vi "1_Boolean_Adder(Training).vi"() -> ()   [LabVIEW 2020]
uses:
  <vilib>/Ngene/DeepLTK/Toolkit/NN_Train/Controls/NN_Train_Params.ctl
  <vilib>/Ngene/DeepLTK/Toolkit/NN_Train/Controls/NN_Train_Optimizer.ctl
  <vilib>/Ngene/DeepLTK/Toolkit/NN_Train/Controls/NN_Train_Data_Sampling.ctl
  <vilib>/Ngene/DeepLTK/Toolkit/NN_Train/Controls/NN_LR_Policy_Cfg.ctl
  <vilib>/Ngene/DeepLTK/Toolkit/NN_Train/Controls/NN_LR_Policy_Type.ctl
  <vilib>/Ngene/DeepLTK/Toolkit/NN_Train/Controls/NN_Train_Session_Data.ctl
  <vilib>/Ngene/DeepLTK/Toolkit/NN_Data/API/DataSet_Types/NN_DataSet(In1D_Out1D).ctl
  <vilib>/Ngene/DeepLTK/Toolkit/NN_Data/API/DataRef_Types/NN_Data_ref(2D_SGL).ctl
  <vilib>/Ngene/DeepLTK/Toolkit/NN_Data/API/DataRef_Types/NN_Data_ref(1D_I32).ctl
  <vilib>/Ngene/DeepLTK/Toolkit/NN_Network/Controls/NN_Device.ctl
  <vilib>/Ngene/DeepLTK/Toolkit/NN_Layers/Layers/FC/Controls/NN_Layer_Config(FC).ctl
  <vilib>/Ngene/DeepLTK/Toolkit/NN_Activations/Controls/NN_Activation_Type.ctl
  <vilib>/Ngene/DeepLTK/Toolkit/NN_Layers/Controls/NN_Layer_Init_Params.ctl
  <vilib>/Ngene/DeepLTK/Toolkit/NN_Layers/Controls/NN_Layer_Weight_Init_Type.ctl
  <vilib>/Ngene/DeepLTK/Toolkit/NN_Network/Controls/NN_Save_Before_Destroy_Options.ctl
  <vilib>/Ngene/DeepLTK/Toolkit/NN_Layers/Layers/Input/Controls/NN_Layer_Config(Input1D).ctl
  <vilib>/Ngene/DeepLTK/Toolkit/NN_Layers/Layers/Input/NN_Layer_Create(Input1D).vi
  <vilib>/Ngene/DeepLTK/Toolkit/NN_Layers/Layers/FC/NN_Layer_Create(FC).vi
  <vilib>/Ngene/DeepLTK/Toolkit/NN_Train/Loss_Functions/NN_Set_Loss(MSE).vi
  <vilib>/Ngene/DeepLTK/Toolkit/NN_Network/subVIs/NN_Predict/NN_Predict(In1D_Out1D).vi
  <vilib>/Ngene/DeepLTK/Toolkit/Deep_Learning_Toolkit_by_Ngene.lvlib
  <vilib>/ptbypt/NI_PtbyPt.lvlib
panel:
  out "Loss Chart":cluster{"mean":dbl, "Error Rate":dbl}(graph)={"mean"=0.0016345112270209938, "Error Rate"=0.0}
  in  "stop":bool
  out "Loop Time":dbl=0.31297880000056466 format="%#_4p"
  out "Error Rate":dbl format="%#_6p"
  out "Loss":sgl=0.0016345113 format="%#_6p"
  in  "?":bool=TRUE
  out "Session Data":T1={"Epochs"=6.9160156, "Tot_Iter"=7082, "LR"=0.05, "LR_iter"=7083}
  in  "LR_Decay_Params":T2={"Policy_Type"=enum."Step", "LR0"=0.09999999999999999, "k"=5.0, "WarmUp_Policy"=enum."Ramp", "WarmUp_Iter"=1000, "WarmUp_Ratio"=1000.0} {"WarmUp_Ratio" min=1; "WarmUp_Iter" min=1; "LR0" format="%.7f"}
  in  "NN_Train_Params":T4={"Optimizer"=enum."SGD", "Beta_1"=0.9, "Beta_2"=0.0, "Weight Decay(L1)"=1e-08, "Weight Decay(L2)"=1e-08, "Data_Sampling"=enum."Random"}
  # "Overview: Demonstrates the usage of Deep Learning Toolkit for solving Boolean Adder problem.\nRequirements: DeepLTK - Deep Learning Toolkit for LabVIEW (https://www.ngene.co/deep-learning-toolkit-for-labview)\nInstructions:\n1. Run the VI.\n2. Observe how the training loss is decreasing.\n3. Observe the training speed.\n4. Press the Stop Train button when the curve stops decreasing.\nMore Examples:  https://github.com/ngenehub/deepltk_examples"
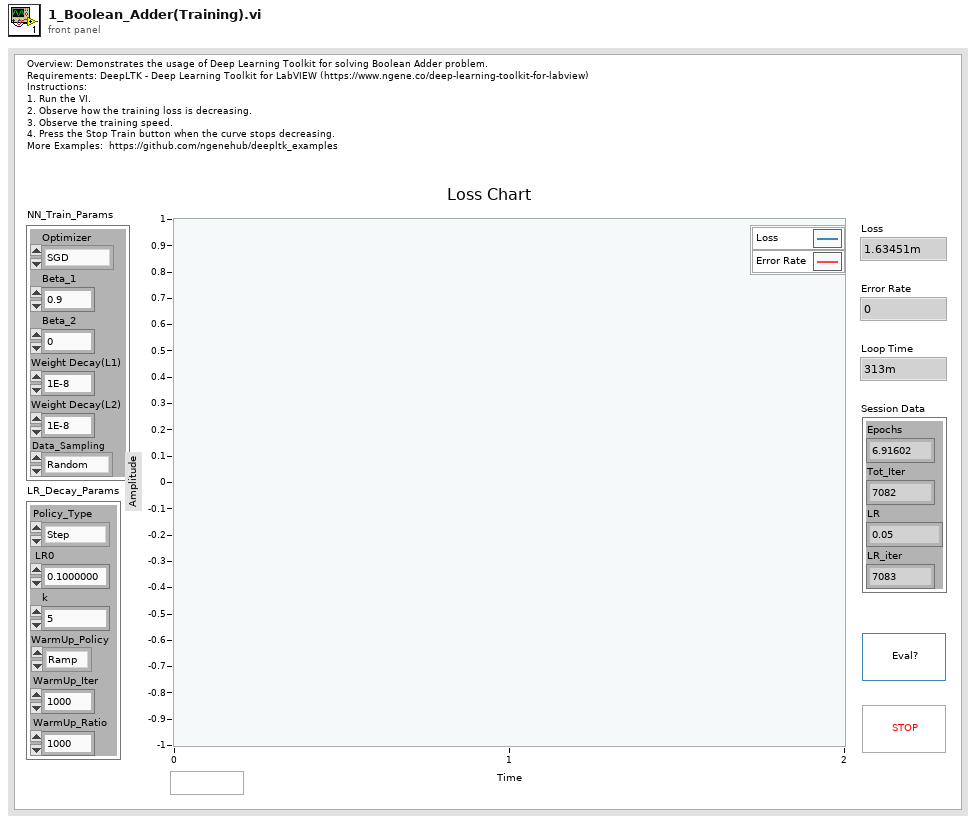
[diagram p1: front panel]
types:
  T1 = typedef "Deep_Learning_Toolkit_by_Ngene.lvlib/NN_Train_Session_Data.ctl" = cluster{"Epochs":sgl, "Tot_Iter":i32, "LR":sgl, "LR_iter":i32}
  T2 = typedef "Deep_Learning_Toolkit_by_Ngene.lvlib/NN_LR_Policy_Cfg.ctl" = cluster{"Policy_Type":T3, "LR0":dbl, "k":sgl, "WarmUp_Policy":enum16{"Step", "Ramp"}, "WarmUp_Iter":i32, "WarmUp_Ratio":sgl}
  T3 = typedef "Deep_Learning_Toolkit_by_Ngene.lvlib/NN_LR_Policy_Type.ctl" = enum16{"Manual", "Step", "Exp", "1/t"}
  T4 = typedef "Deep_Learning_Toolkit_by_Ngene.lvlib/NN_Train_Params.ctl" = cluster{"Optimizer":T5, "Beta_1":sgl, "Beta_2":sgl, "Weight Decay(L1)":sgl, "Weight Decay(L2)":sgl, "Data_Sampling":T6}
  T5 = typedef "Deep_Learning_Toolkit_by_Ngene.lvlib/NN_Train_Optimizer.ctl" = enum16{"SGD", "Adam", "Adagrad", "Adadelta", "RMSProp", "Nesterov"}
  T6 = typedef "Deep_Learning_Toolkit_by_Ngene.lvlib/NN_Train_Data_Sampling.ctl" = enum16{"Random", "Sequential"}
  T7 = typedef "Deep_Learning_Toolkit_by_Ngene.lvlib/NN_DataSet(In1D_Out1D).ctl" = cluster{"Inputs Ref.":T8, "Outputs Ref.":T8, "Dims_In":i32, "Dataset_Size":i32, "Outputs_idx Ref.":T9, "Dims_Out":i32, "Labels":string[], "File Paths":path[]}
  T8 = typedef "Deep_Learning_Toolkit_by_Ngene.lvlib/NN_Data_ref(2D_SGL).ctl" = refnum<data-value>
  T9 = typedef "Deep_Learning_Toolkit_by_Ngene.lvlib/NN_Data_ref(1D_I32).ctl" = refnum<data-value>
  T10 = typedef "Deep_Learning_Toolkit_by_Ngene.lvlib/NN_Layer_Config(FC).ctl" = cluster{"Name":string, "Size":i32, "BN":bool, "Activation":T11, "Init_Params":T12, "Custom_Params":string}
  T11 = typedef "Deep_Learning_Toolkit_by_Ngene.lvlib/NN_Activation_Type.ctl" = enum16{"Sigmoid", "ReLU", "LReLU", "ReLU6", "tanh", "Swish", "Mish", "None"}
  T12 = typedef "Deep_Learning_Toolkit_by_Ngene.lvlib/NN_Layer_Init_Params.ctl" = cluster{"Init_Type":T13, "Value":sgl}
  T13 = typedef "Deep_Learning_Toolkit_by_Ngene.lvlib/NN_Layer_Weight_Init_Type.ctl" = enum16{"Const", "Uniform", "Gaussian", "Xavier"}
  T14 = typedef "Deep_Learning_Toolkit_by_Ngene.lvlib/NN_Device.ctl" = enum16{"CPU", "GPU"}
  T15 = typedef "Deep_Learning_Toolkit_by_Ngene.lvlib/NN_Save_Before_Destroy_Options.ctl" = cluster{"CFG?":bool, "Weights?":bool, "Render?":bool}
  T16 = typedef "Deep_Learning_Toolkit_by_Ngene.lvlib/NN_Layer_Config(Input1D).ctl" = cluster{"Name":string, "Size":i32}
  T17 = typedef "Deep_Learning_Toolkit_by_Ngene.lvlib/NN.ctl" = cluster{"Name":string, "No of Layers":i32, "mBatch":i32, "Layers":T18[], "Dimty":T19, "Dims_In":T20, "Dims_Out":T20, "Working_Dir":path, "Train?":bool, "Train_Params":T4, "LR_Update_Policy":T2, "Session Data":T1, "Ground_truth":T21, "NNg_hdls":T22, "NN_Device":T14, "GPU Id":i32, "Labels":string[], "Receptive Field":T23[], "Loss_Type":T24, "Loss_Cfg_Prms":variant}
  T18 = typedef "Deep_Learning_Toolkit_by_Ngene.lvlib/NN_Layer_ref.ctl" = refnum<data-value>
  T19 = typedef "Deep_Learning_Toolkit_by_Ngene.lvlib/NN_In_Out_Dim-ty.ctl" = enum8{"In1D_Out1D", "In3D_Out1D", "In3D_Out3D", "In3D_OutBBox"}
  T20 = typedef "Deep_Learning_Toolkit_by_Ngene.lvlib/NN_Dims(C,H,W).ctl" = cluster{"C":i32, "H":i32, "W":i32}
  T21 = typedef "Deep_Learning_Toolkit_by_Ngene.lvlib/NN_Ground_truth.ctl" = cluster{"Y":variant, "Y_idx":T9}
  T22 = typedef "Deep_Learning_Toolkit_by_Ngene.lvlib/nng_cuda_handles.ctl" = cluster{"cudnn":u64, "cublas":u64, "stream":u64, "curand":u64}
  T23 = typedef "Deep_Learning_Toolkit_by_Ngene.lvlib/NN_Dims(V,H).ctl" = cluster{"V":i32, "H":i32}
  T24 = typedef "Deep_Learning_Toolkit_by_Ngene.lvlib/NN_Loss_Type.ctl" = enum16{"None", "MSE", "CrossEntropy", "YOLO_v2"}
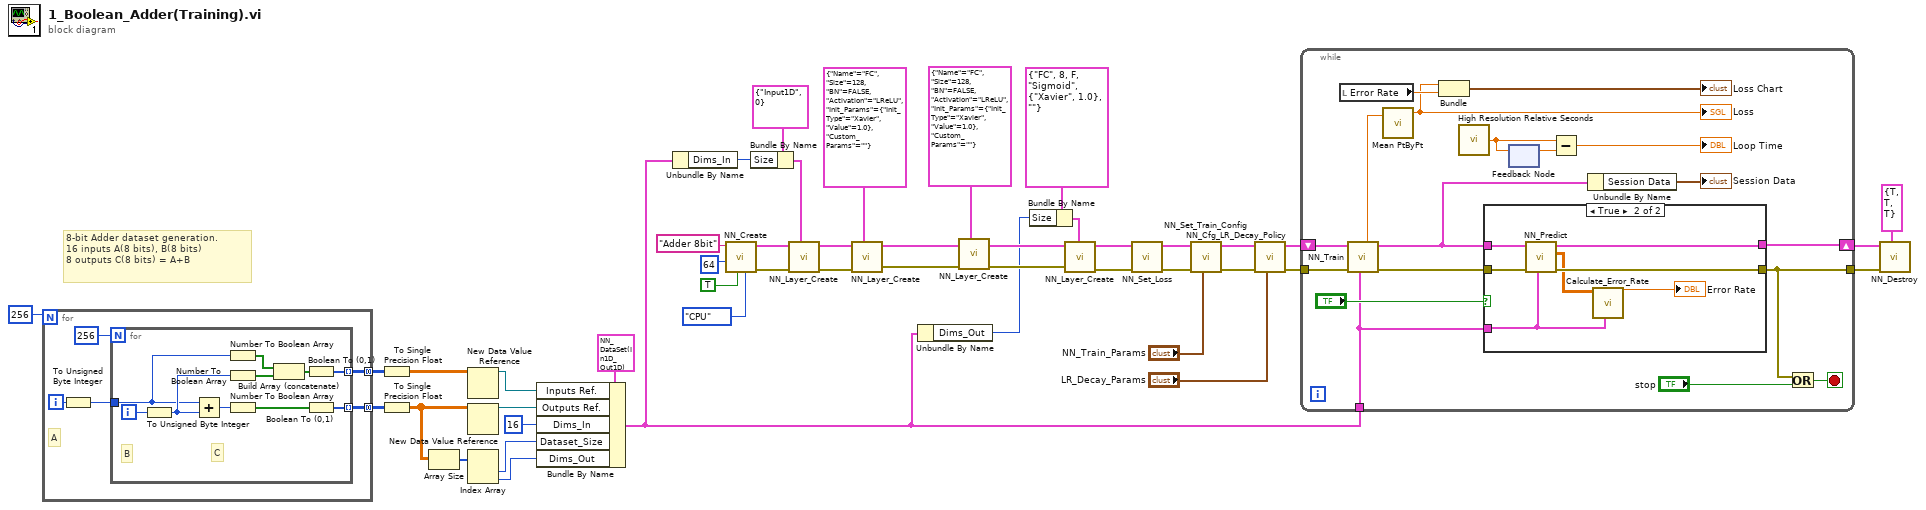
[diagram p0: block diagram]
diagram:
  # "8-bit Adder dataset generation.\n16 inputs A(8 bits), B(8 bits)\n8 outputs C(8 bits) = A+B"
  n1 = for {
    N: 256 -> [_]
    tunnel: [w50] -> w14 mode=concatenating
    tunnel: [w49] -> w13 mode=concatenating
    i -> [w48]
    # "A"
    n2 = To Unsigned Byte Integer(number=w48) -> (unsigned 8bit integer=w47:u8)
    n3 = for {
      N: 256 -> [_]
      tunnel: [w60] -> w49 mode=indexing
      tunnel: [w57] -> w50 mode=indexing
      tunnel: w47 -> [w54]
      i -> [w56]
      # "C"
      # "B"
      n4 = To Unsigned Byte Integer(number=w56) -> (unsigned 8bit integer=w55:u8)
      n5 = Add(x=w54, y=w55) -> (x+y=w58:u8)
      n6 = Number To Boolean Array(number=w54) -> (Boolean array=w52:bool[])
      n7 = Number To Boolean Array(number=w55) -> (Boolean array=w61:bool[])
      n8 = Number To Boolean Array(number=w58) -> (Boolean array=w59:bool[])
      n9 = Build Array (concatenate)(w52, w61) -> (w53:bool[])
      n10 = Boolean To (0,1)(Boolean=w53) -> (0, 1=w60:i16[])
      n11 = Boolean To (0,1)(Boolean=w59) -> (0, 1=w57:i16[])
    }
  }
  n12 = To Single Precision Float(number=w13) -> (single precision float=w7:sgl[][])
  n13 = To Single Precision Float(number=w14) -> (single precision float=w11:sgl[][])
  n14 = Array Size(array=w11) -> (size(s)=w10:i32[])
  n15 = New Data Value Reference(data value=w7) -> (data value reference=w16:refnum<data-value>)  [unwired: 1 in, 1 out]
  n16 = New Data Value Reference(data value=w11) -> (data value reference=w15:refnum<data-value>)  [unwired: 1 in, 1 out]
  n17 = Index Array(array=w10) -> (element #1=w9:i32, element #2=w8:i32)  [unwired: 2 in]
  n18 = Bundle By Name(cluster=T7 {"Inputs Ref."=refnum, "Outputs Ref."=refnum, "Dims_In"=0, "Dataset_Size"=0, "Outputs_idx Ref."=refnum, "Dims_Out"=0, "Labels"=[], "File Paths"=[]} ("Dataset(In1D_Out1D)"), "Inputs Ref."=w16, "Outputs Ref."=w15, "Dims_In"=16, "Dataset_Size"=w9, "Dims_Out"=w8) -> (w1:T7)
  n19 = Unbundle By Name(w1) -> ("Dims_In"=w2:i32)
  n20 = call <vilib>:"NN_Create.vi"("NN_Device"=NN_Device."CPU", "Train? (false)"=TRUE, "mBatch (1)"=64, "Name"="Adder 8bit") -> ("error out"=w43:errorcluster, "NN out"=w44:T17)  [unwired: 6 in]
  n21 = Bundle By Name(cluster=T16 {"Name"="Input1D", "Size"=0} ("Input1D_Cfg"), "Size"=w2) -> (w38:T16)
  n22 = call-poly <vilib>:"NN_Layer_Create.vi"("Input1D_Cfg"=w38, "error in (no error)"=w43, "NN in"=w44) -> ("error out"=w46:errorcluster, "NN out"=w45:T17)  [unwired: 6 in, 1 out]
  n23 = call-poly <vilib>:"NN_Layer_Create.vi"("FC_Cfg"=T10 {"Name"="FC", "Size"=128, "BN"=FALSE, "Activation"=enum."LReLU", "Init_Params"={"Init_Type"=enum."Xavier", "Value"=1.0}, "Custom_Params"=""}, "error in (no error)"=w46, "NN in"=w45) -> ("error out"=w20:errorcluster, "NN out"=w21:T17)  [unwired: 6 in, 1 out]
  n24 = Unbundle By Name(w1) -> ("Dims_Out"=w3:i32)
  n25 = call-poly <vilib>:"NN_Layer_Create.vi"("FC_Cfg"=T10 {"Name"="FC", "Size"=128, "BN"=FALSE, "Activation"=enum."LReLU", "Init_Params"={"Init_Type"=enum."Xavier", "Value"=1.0}, "Custom_Params"=""}, "error in (no error)"=w20, "NN in"=w21) -> ("error out"=w19:errorcluster, "NN out"=w18:T17)  [unwired: 6 in, 1 out]
  n26 = Bundle By Name(cluster=T10 {"Name"="FC", "Size"=8, "BN"=FALSE, "Activation"=enum."Sigmoid", "Init_Params"={"Init_Type"=enum."Xavier", "Value"=1.0}, "Custom_Params"=""} ("FC_Cfg"), "Size"=w3) -> (w4:T10)
  n27 = call-poly <vilib>:"NN_Layer_Create.vi"("FC_Cfg"=w4, "error in (no error)"=w19, "NN in"=w18) -> ("error out"=w24:errorcluster, "NN out"=w23:T17)  [unwired: 6 in, 1 out]
  n28 = call-poly <vilib>:"NN_Set_Loss.vi"("error in (no error)"=w24, "NN in"=w23) -> ("error out"=w25:errorcluster, "NN out"=w26:T17)  [unwired: 8 in]
  n29 = call <vilib>:"NN_Set_Train_Config.vi"("NN_Train_Params"="NN_Train_Params", "error in (no error)"=w25, "NN in"=w26) -> ("error out"=w31:errorcluster, "NN out"=w36:T17)  [unwired: 7 in]
  n30 = call <vilib>:"NN_Cfg_LR_Decay_Policy.vi"("LR_Decay_Params"="LR_Decay_Params", "error in (no error)"=w31, "NN in"=w36) -> ("error out"=w30:errorcluster, "NN out"=w32:T17)  [unwired: 7 in]
  n31 = while {
    tunnel: w30 -> [w78]
    tunnel: w1 -> [w70]
    shift-right: [w74] -> w34
    shift-left: w32 -> [w79]
    tunnel: [w69] -> w33
    stop <- w64 stop-if-true
    n32 = local read "Error Rate"() -> (w71:dbl)
    n33 = call <vilib>:"NN_Train.vi"("Train Dataset"=w70, "error in (no error)"=w78, "NN in"=w79) -> ("error out"=w73:errorcluster, "NN out"=w76:T17, "Loss"=w77:sgl)  [unwired: 5 in, 1 out]
    n34 = call <vilib>:"Mean PtByPt.vi"("x"=w77) -> ("mean"=w68:dbl)  [unwired: 3 in, 1 out]
    "Loss" <- w68
    n35 = Bundle("mean"=w68, "Error Rate"=w71) -> (→"Loss Chart":cluster{"mean":dbl, "Error Rate":dbl})  [unwired: 1 in]
    n36 = call <vilib>:"High Resolution Relative Seconds.vi"() -> ("relative seconds"=w66:dbl)
    n37 = case shown="True" "?" {
      tunnel: w76 -> [w81 w86]
      tunnel: [w81 w88] -> w74
      tunnel: w73 -> [w80 w85]
      tunnel: [w80 w87] -> w69
      tunnel: w70 -> [_ w82]
      frame False {
      }
      frame True {
        n38 = call-poly <vilib>:"NN_Predict.vi"("Dataset"=w82, "error in (no error)"=w85, "NN in"=w86) -> ("error out"=w87:errorcluster, "Predictions"=w84:sgl[][], "NN out"=w88:T17)  [unwired: 6 in]
        n39 = call "Calculate_Error_Rate.vi"("Dataset(In1D_Out1D)"=w82, "Predictions"=w84) -> ("Error Rate"=→"Error Rate":dbl)  [unwired: 9 in]
      }
    }
    n40 = feedback #1() -> (w65:dbl)  [unwired: 1 in]
    n41 = feedback-in #1(w66) -> ()
    n42 = Subtract(x=w66, y=w65) -> (x-y=→"Loop Time":dbl)
    n43 = Unbundle By Name(w76) -> ("Session Data"=→"Session Data":T1)
    n44 = Or(x=w69, y="stop") -> (x .or. y?=w64:bool)
  }
  n45 = call <vilib>:"NN_Destroy.vi"("Save (T, T, T)"=T15 {"CFG?"=TRUE, "Weights?"=TRUE, "Render?"=TRUE}, "error in (no error)"=w33, "NN in"=w34) -> ()  [unwired: 8 in, 1 out]
